vi "Elevator Controller.vi"(8 "error in":errorcluster) -> ()   [LabVIEW 2017]
doc: "This VI executes continuously carrying out the current operation and responding to updates or new operations. It will often contain the timing or control code that is difficult to place directly in TeleOp. This VI generally opens all sensors and motors and isolates the rest of the robot code from knowing how the operations are carried out."
uses:
  <vilib>/Rock Robotics/WPI/Framework/Completion Status.ctl
  Elevator Setpoints.ctl
  Elevator Operations.ctl
  Private/Typedef/Sequencer State Data.ctl
  Private/Typedef/Sequencer States.ctl
panel:
  in  "Interactive Values":T1
  out "Current\nCmd":string
  in  "Buttons":cluster{"Execute Cmd":bool, "Abort Cmd":bool}
  out "Command Timing":cluster{"Start Time (ms)":u32, "Iterations":i32}
  out "Status":T3
  # "Tip: It may be helpful to observe inputs and sensor values.\nYou may also want to display tuning or debugging controls."
  # "Interactive Command: You may fill in the settings for a command\nand schedule it with the Execute button. You can observe and abort\nany command while fine tuning the code for the controller."
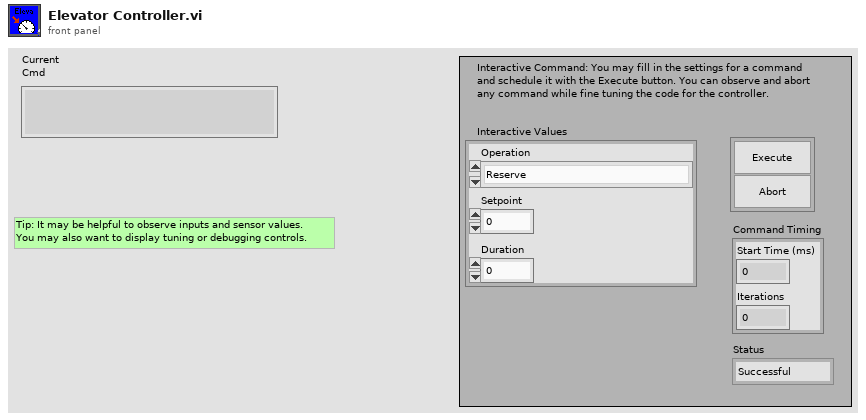
[diagram p1: front panel]
types:
  T1 = typedef "Elevator Setpoints.ctl" = cluster{"Operation":T2, "Setpoint":dbl, "Duration":dbl}
  T2 = typedef "Elevator Operations.ctl" = enum16{"Reserve", "Read Current", "Immediate", "Stop", "Pickup", "Switch", "Scale", "Manual Up", "Manual Down", "Home"}
  T3 = typedef "Completion Status.ctl" = enum16{"Successful", "Aborted", "Incomplete"}
  T4 = cluster{"Elevator":refnum<notifier>, "Gripper":refnum<notifier>}
  T5 = typedef "Sequencer State Data.ctl" = cluster{"State":T6, "Data":dbl}
  T6 = typedef "Sequencer States.ctl" = enum16{"Init", "Set Elevator SP", "Set Gripper SP", "Wait For Elevator", "Wait For Gripper", ""}
  T7 = typedef "Command Status Info.ctl" = cluster{"Name":string, "Status":T3, "notifier out":T8}
  T8 = typedef "Completion Notifier.ctl" = refnum<notifier>
  T9 = cluster{"Current Command":T1, "Command Timing":cluster{"Start Time (ms)":u32, "Iterations":i32}, "Command Arguments":cluster{"Command Info":T7, "Description":string, "Default Command":T1, "queue out":refnum<queue>, "Subsystem Name":string}}
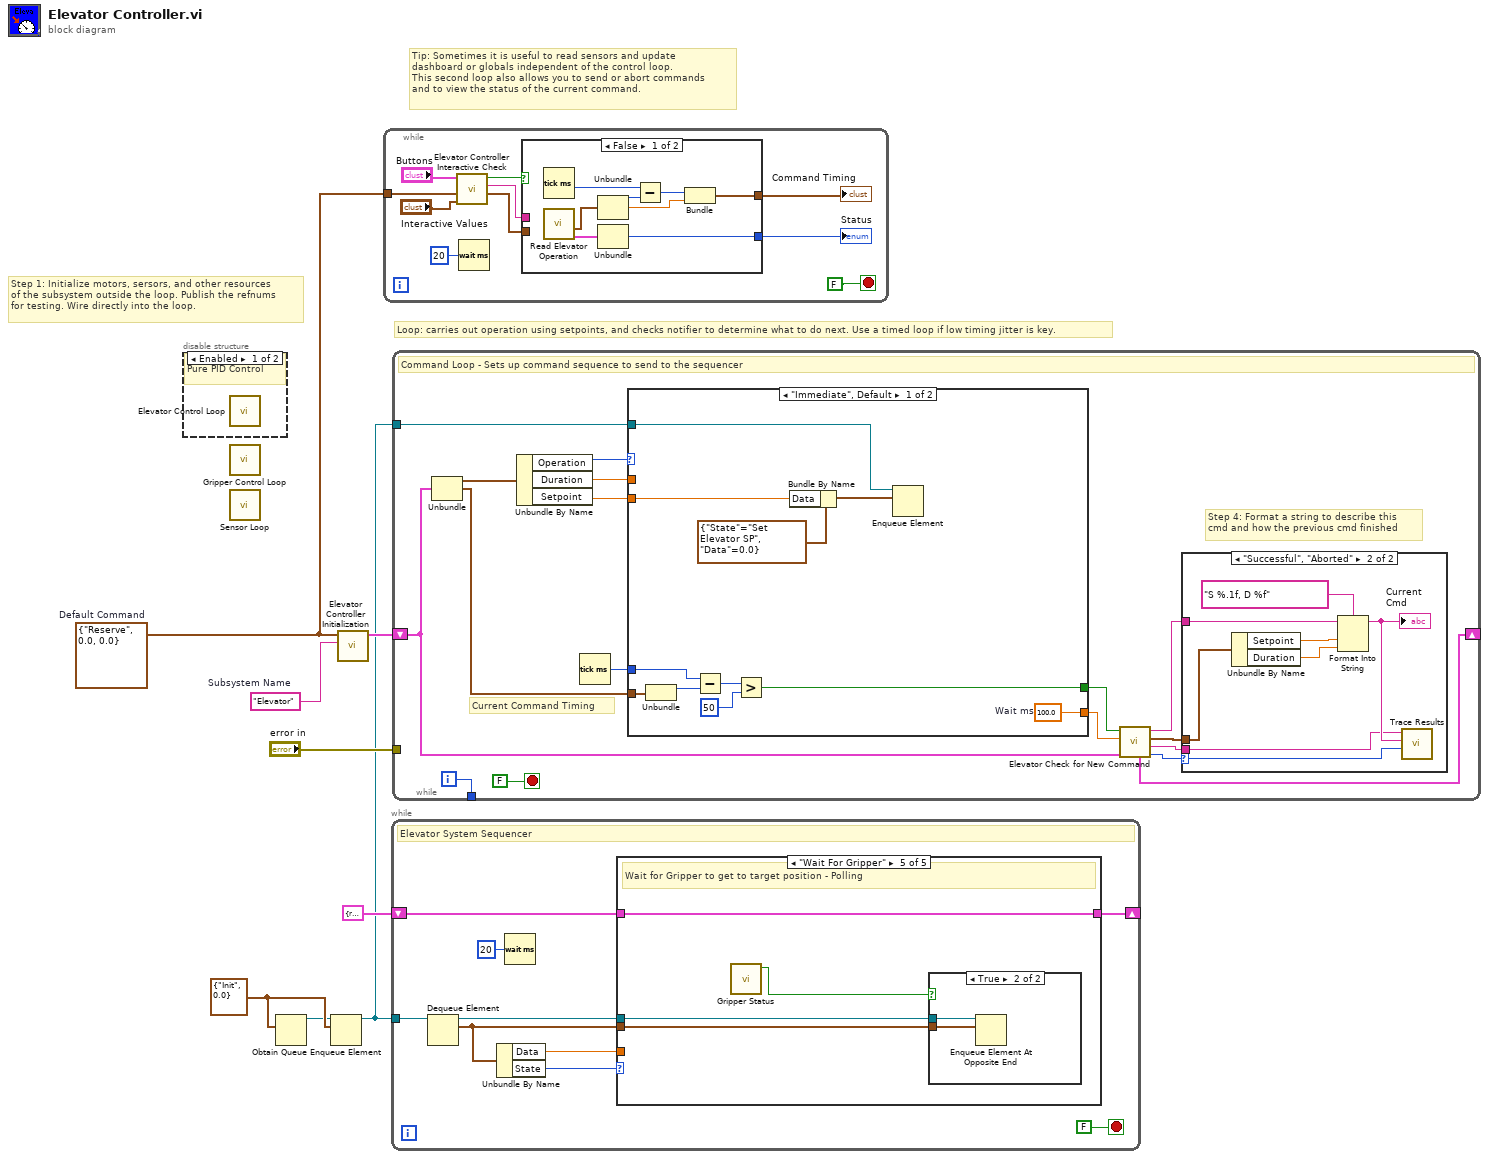
[diagram p0: block diagram]
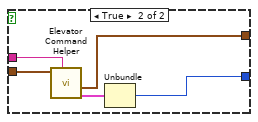
[diagram p2: hidden frame]
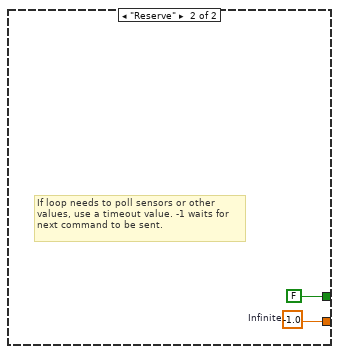
[diagram p3: hidden frame]
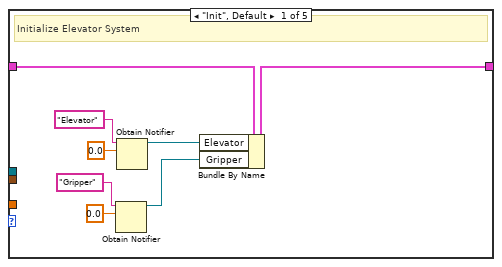
[diagram p5: hidden frame]
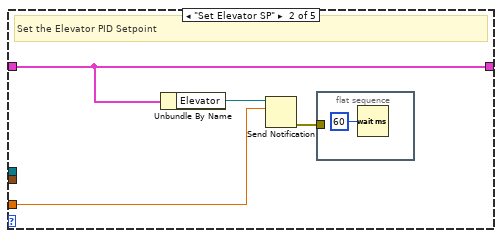
[diagram p6: hidden frame]
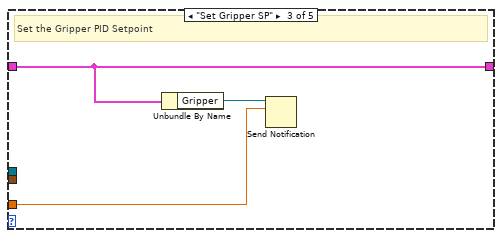
[diagram p7: hidden frame]
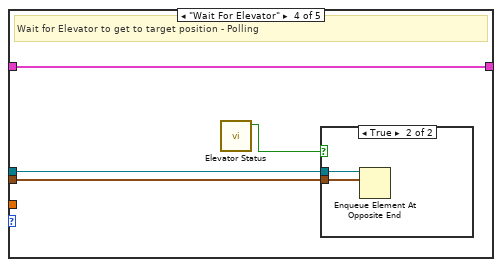
[diagram p8: hidden frame]
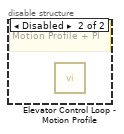
[diagram p11: hidden frame]
diagram:
  w3 = T5 {"State"=enum."Init", "Data"=0.0}
  w5 = T1 {"Operation"=enum."Reserve", "Setpoint"=0.0, "Duration"=0.0}  # Default Command
  w6 = "Elevator"  # Subsystem Name
  # "Tip: Sometimes it is useful to read sensors and update\ndashboard or globals independent of the control loop.\nThis second loop also allows you to send or abort commands\nand to view the status of the current command."
  # "Step 1: Initialize motors, sersors, and other resources\nof the subsystem outside the loop. Publish the refnums\nfor testing. Wire directly into the loop."
  # "Loop: carries out operation using setpoints, and checks notifier to determine what to do next. Use a timed loop if low timing jitter is key."
  n1 = disable-structure shown="Enabled" {
    frame Enabled {
      # "Pure PID Control"
      n2 = call "Elevator Control Loop.vi"() -> ()  [unwired: 12 in]
    }
    frame Disabled {
      # "Motion Profile + PI"
      n3 = call "Elevator Control Loop - Motion Profile.vi"() -> ()  [unwired: 12 in]
    }
  }
  n4 = call "Gripper Control Loop.vi"() -> ()  [unwired: 12 in]
  n5 = call "Sensor Loop.vi"() -> ()  [unwired: 12 in]
  n6 = Obtain Queue(element data type=w3) -> (queue out=w2:refnum<queue>)  [unwired: 4 in, 2 out]
  n7 = Enqueue Element(queue=w2, element=w3) -> (queue out=w1:refnum<queue>)  [unwired: 2 in, 2 out]
  n8 = call "Elevator Controller Initialization.vi"("Subsystem Name"=w6, "Default Command"=w5) -> ("Current Command"=w7:T9)  [unwired: 9 in]
  n9 = while {
    tunnel: w5 -> [w15]
    stop <- FALSE stop-if-true
    n10 = call "Elevator Controller Interactive Check.vi"("Interactive Command in"="Interactive Values", "Default Command"=w15, "Buttons"="Buttons") -> ("Interactive Command out"=w12:T1, "Trace String"=w13:string, "Schedule"=w14:bool)  [unwired: 6 in]
    n11 = Wait (ms)(milliseconds to wait=u32 20) -> ()  [unwired: 1 out]
    n12 = case shown="False" w14 {
      tunnel: [w26 w31] -> w11
      tunnel: w12 -> [_ w29]
      tunnel: [w22 w27] -> w10
      tunnel: w13 -> [_ w30]
      frame False {
        n13 = Tick Count (ms)() -> (millisecond timer value=w21:u32)
        n14 = call "Read Elevator Operation.vi"() -> ("Command Info"=w19:T7, "SubSystem Data"=w20:T1)  [unwired: 9 in, 1 out]
        n15 = Unbundle(w20) -> ("Operation"=w25:T2, "Setpoint"=w23:dbl)  [unwired: 1 out]
        n16 = Unbundle(w19) -> ("Status"=w26:T3)  [unwired: 2 out]
        n17 = Subtract(x=w21, y=w25) -> (x-y=w24:u32)
        n18 = Bundle(w24, "Setpoint"=w23) -> (w22:cluster{u32, "Setpoint":dbl})  [unwired: 1 in]
      }
      frame True {
        n19 = call "Elevator Command Helper.vi"("Description"=w30, "SubSystem Data"=w29) -> ("Command Info Out"=w28:T7, "Command Timing"=w27:cluster{"Start Time (ms)":u32, "Iterations":i32})  [unwired: 7 in, 1 out]
        n20 = Unbundle(w28) -> ("Status"=w31:T3)  [unwired: 2 out]
      }
    }
    "Status" <- w11
    "Command Timing" <- w10
  }
  n21 = while {
    tunnel: w1 -> [w38]
    shift-right: [w33] -> _
    shift-left: T4 {"Elevator"=refnum, "Gripper"=refnum} -> [w34]
    stop <- FALSE stop-if-true
    # "Elevator System Sequencer"
    n22 = Dequeue Element(queue=w38) -> (queue out=w37:refnum<queue>, element=w32:T5)  [unwired: 2 in, 2 out]
    n23 = Unbundle By Name(w32) -> ("Data"=w35:dbl, "State"=w36:T6)
    n24 = Wait (ms)(milliseconds to wait=u32 20) -> ()  [unwired: 1 out]
    n25 = case shown="\"Wait For Gripper\"" w36 {
      tunnel: w37 -> [_ _ _ w59 w64]
      tunnel: w35 -> [_ w50 w54 _ _]
      tunnel: w34 -> [w45 w52 w56 w60 w66]
      tunnel: [w44 w52 w56 w60 w66] -> w33
      tunnel: w32 -> [_ _ _ w58 w65]
      frame "Init", Default {
        # "Initialize Elevator System"
        n26 = Obtain Notifier(name (unnamed)="Gripper", notification data type=0.0 ("Setpoint")) -> (notifier out=w41:refnum<notifier>)  [unwired: 2 in, 2 out]
        n27 = Obtain Notifier(name (unnamed)="Elevator", notification data type=0.0 ("Setpoint")) -> (notifier out=w46:refnum<notifier>)  [unwired: 2 in, 2 out]
        n28 = Bundle By Name(cluster=w45, "Elevator"=w46, "Gripper"=w41) -> (w44:T4)
      }
      frame "Set Elevator SP" {
        # "Set the Elevator PID Setpoint"
        n29 = Unbundle By Name(w52) -> ("Elevator"=w51:refnum<notifier>)
        n30 = Send Notification(notification=w50, notifier=w51) -> (error out=w49:errorcluster)  [unwired: 1 in, 1 out]
        n31 = flat-sequence {
          tunnel: w49 -> [_]
          frame #0 {
            n32 = Wait (ms)(milliseconds to wait=u32 60) -> ()  [unwired: 1 out]
          }
        }
      }
      frame "Set Gripper SP" {
        # "Set the Gripper PID Setpoint"
        n33 = Unbundle By Name(w56) -> ("Gripper"=w55:refnum<notifier>)
        n34 = Send Notification(notification=w54, notifier=w55) -> ()  [unwired: 1 in, 2 out]
      }
      frame "Wait For Elevator" {
        # "Wait for Elevator to get to target position - Polling"
        n35 = call "Elevator Status.vi"() -> ("Moving?"=w57:bool)  [unwired: 9 in, 2 out]
        n36 = case shown="True" w57 {
          tunnel: w59 -> [_ w62]
          tunnel: w58 -> [_ w61]
          frame False {
          }
          frame True {
            n37 = Enqueue Element At Opposite End(queue=w62, element=w61) -> ()  [unwired: 2 in, 3 out]
          }
        }
      }
      frame "Wait For Gripper" {
        # "Wait for Gripper to get to target position - Polling"
        n38 = call "Gripper Status.vi"() -> ("Moving?"=w63:bool)  [unwired: 9 in, 2 out]
        n39 = case shown="True" w63 {
          tunnel: w64 -> [_ w68]
          tunnel: w65 -> [_ w67]
          frame False {
          }
          frame True {
            n40 = Enqueue Element At Opposite End(queue=w68, element=w67) -> ()  [unwired: 2 in, 3 out]
          }
        }
      }
    }
  }
  n41 = while {
    shift-right: [w77] -> _
    shift-left: w7 -> [w70]
    tunnel: [w84] -> _
    tunnel: "error in" -> [_]
    tunnel: w1 -> [w69]
    i -> [w84]
    stop <- FALSE stop-if-true
    # "Step 4: Format a string to describe this\ncmd and how the previous cmd finished"
    # "Current Command Timing"
    # "Command Loop - Sets up command sequence to send to the sequencer"
    n42 = Unbundle(w70) -> ("Current Command"=w83:T1, "Command Timing"=w79:cluster{"Start Time (ms)":u32, "Iterations":i32})  [unwired: 1 out]
    n43 = Unbundle By Name(w83) -> ("Operation"=w82:T2, "Duration"=w81:dbl, "Setpoint"=w78:dbl)
    n44 = Tick Count (ms)() -> (millisecond timer value=w80:u32)
    n45 = case shown="\"Immediate\", Default" w82 {
      tunnel: [w96 w98] -> w75
      tunnel: [w90 FALSE ("ignore previous (F)")] -> w76
      tunnel: w79 -> [w92 _]
      tunnel: w81 -> [_ _]
      tunnel: w80 -> [w91 _]
      tunnel: w78 -> [w86 _]
      tunnel: w69 -> [w89 _]
      frame "Immediate", Default {
        w96 = 100.0  # Wait ms
        n46 = Unbundle(w92) -> ("Start Time (ms)"=w95:u32)  [unwired: 1 out]
        n47 = Subtract(x=w91, y=w95) -> (x-y=w94:u32)
        n48 = Greater?(x=w94, y=u8 50 ("Left Motor")) -> (0:w90:bool)
        n49 = Bundle By Name(cluster=T5 {"State"=enum."Set Elevator SP", "Data"=0.0} ("element"), "Data"=w86) -> (w88:T5)
        n50 = Enqueue Element(queue=w89, element=w88) -> ()  [unwired: 2 in, 3 out]
      }
      frame "Reserve" {
        w98 = -1.0  # Infinite
        # "If loop needs to poll sensors or other\nvalues, use a timeout value. -1 waits for\nnext command to be sent."
      }
    }
    n51 = call "Elevator Check for New Command.vi"("Current Command"=w70, "Wait time (ms)"=w75, "Finished?"=w76) -> ("Completion"=w71:T3, "Subsystem Name"=w72:string, "Current Command"=w73:T1, "Initial Trace String"=w74:string, "NextCommand"=w77:T9)  [unwired: 4 in]
    n52 = case shown="\"Successful\", \"Aborted\"" w71 {
      selector: w71 -> [_ w106]
      tunnel: w74 -> [_ w102]
      tunnel: w73 -> [_ w103]
      tunnel: w72 -> [_ w99]
      frame "Incomplete", Default {
        # "Continuing current command"
      }
      frame "Successful", "Aborted" {
        # "Report and setup for next command"
        n53 = Unbundle By Name(w103) -> ("Setpoint"=w105:dbl, "Duration"=w100:dbl)
        n54 = Format Into String(format string="S %.1f, D %f", initial string=w102, w105, w100) -> (resulting string=w101:string)  [unwired: 1 in, 1 out]
        "Current\nCmd" <- w101
        n55 = call <vilib>:"Trace Results.vi"("Status of previous command"=w106, "Description"=w101, "Subsystem"=w99) -> ()  [unwired: 9 in]
      }
    }
  }
